vi "Switch tables 2.vi"() -> ()   [LabVIEW 2016]
uses:
  <userlib>/LevyLab/postgreSQL-timescaleDB/Data.PG/Data.PGSQL.lvclass
panel:
  out "Result":string[][](array[string])
  in  "error in (no error)":errorcluster
  out "error out":errorcluster
  in  "New Table":string
  in  "Old  Table":string
  in  "Old Column":string
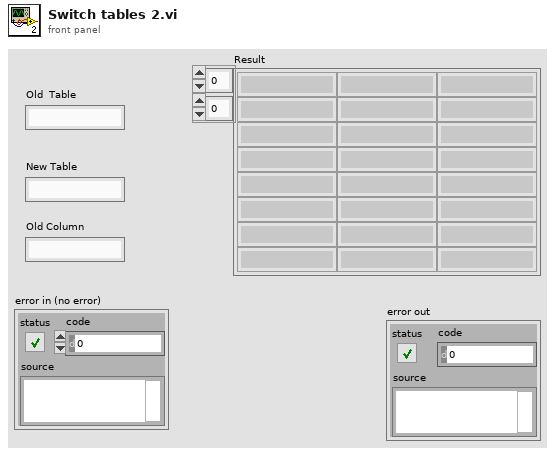
[diagram p1: front panel]
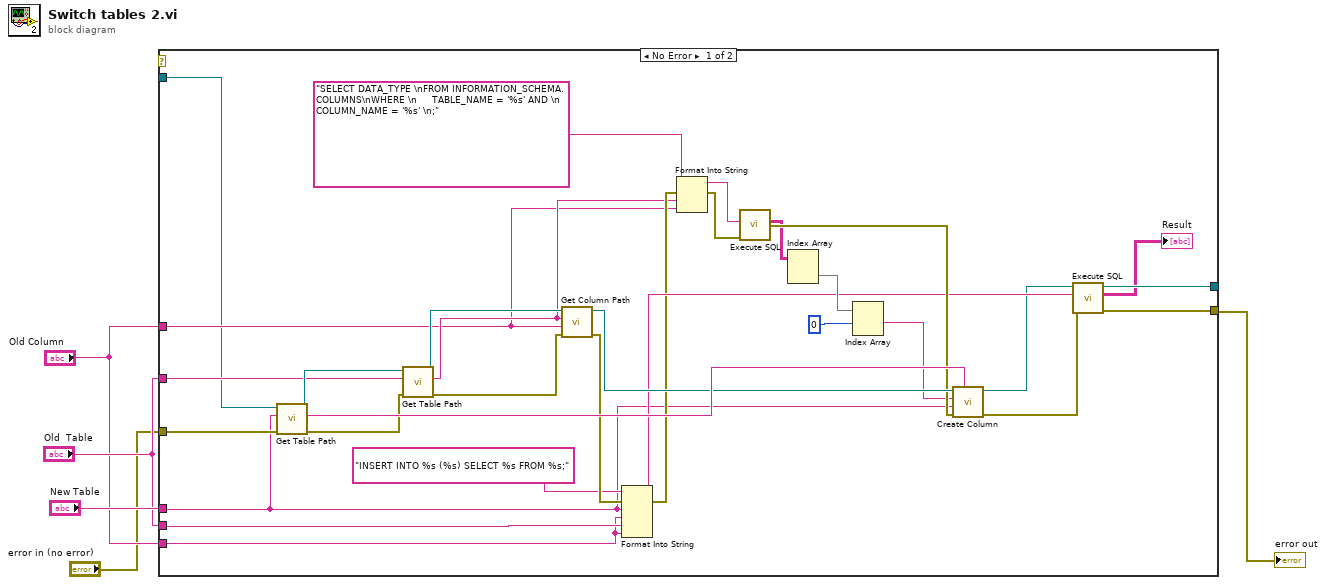
[diagram p0: block diagram]
diagram:
  n1 = case shown="No Error" {
    selector: _ -> [_ _]
    tunnel: "Old  Table" -> [w18 _]
    tunnel: "Old Column" -> [w17 _]
    tunnel: "New Table" -> [w11 _]
    tunnel: "Old  Table" -> [w16 _]
    tunnel: "Old Column" -> [w14 _]
    tunnel: "error in (no error)" -> [w13 w39]
    tunnel: [w12 w40] -> w4
    tunnel: [w10 w39] -> w3
    tunnel: [w9 w40] -> w2
    frame No Error {
      n2 = call <userlib>:"Get Table Path.vi"("error in (no error)"=w13, "Table"=w11, "Data.PG"=w12) -> ("error out"=w24:errorcluster, "Table Path"=w36:string, "Data.PG out"=w23:refnum<class "Data.PGSQL.lvclass">)  [unwired: 6 in]
      n3 = call <userlib>:"Get Table Path.vi"("error in (no error)"=w24, "Table"=w16, "Data.PG"=w23) -> ("error out"=w37:errorcluster, "Table Path"=w15:string, "Data.PG out"=w38:refnum<class "Data.PGSQL.lvclass">)  [unwired: 6 in]
      n4 = call <userlib>:"Get Column Path.vi"("error in (no error)"=w37, "Column"=w14, "Table path"=w15, "Data.PG in"=w38) -> ("error out"=w22:errorcluster, "Data.PG out"=w35:refnum<class "Data.PGSQL.lvclass">)  [unwired: 4 in, 2 out]
      n5 = Format Into String(initial string="INSERT INTO %s (%s) SELECT %s FROM %s;", error in=w22, w11, w17, w18, w17) -> (resulting string=w26:string, error out=w21:errorcluster)  [unwired: 1 in]
      n6 = Format Into String(initial string="SELECT DATA_TYPE \nFROM INFORMATION_SCHEMA.COLUMNS\nWHERE \n     TABLE_NAME = '%s' AND \n     COLUMN_NAME = '%s' \n;", error in=w21, w15, w14) -> (resulting string=w33:string, error out=w20:errorcluster)  [unwired: 1 in]
      n7 = call <userlib>:"Execute SQL.vi"("error in"=w20, "SQL"=w33) -> ("error out"=w32:errorcluster, "Result"=w29:string[][])  [unwired: 7 in, 1 out]
      n8 = Index Array(array=w29) -> (element=w30:string[])  [unwired: 2 in]
      n9 = Index Array(array=w30, index #1=0 ("index")) -> (element #1=w28:string)  [unwired: 1 in, 1 out]
      n10 = call <userlib>:"Create Column.vi"("selected table path"=w36, "error in (no error)"=w32, "new column name"=w11, "new column data type"=w28, "Data.PGSQL in"=w35) -> ("error out"=w27:errorcluster, "Data.PGSQL out"=w25:refnum<class "Data.PGSQL.lvclass">)  [unwired: 5 in]
      n11 = call <userlib>:"Execute SQL.vi"("error in"=w27, "SQL"=w26, "Data.PG"=w25) -> ("error out"=w10:errorcluster, "Result"=→"Result":string[][], "Data.PG out"=w9:refnum<class "Data.PGSQL.lvclass">)  [unwired: 6 in]
    }
    frame Error {
    }
  }
  "error out" <- w3
